vi "echo control.vi"(7 "Read buffer":string="?01E70581\r", 8 "error in":errorcluster) -> (0 "error out":errorcluster, 1 "Сообщение об ошибке":bool, 4 "read buffer wo echo":string, 5 "Ошибка пакета?":bool)   [LabVIEW 2017, in "LV_Unicorn.lvlib"]
uses:
  LV_Unicorn.lvlib
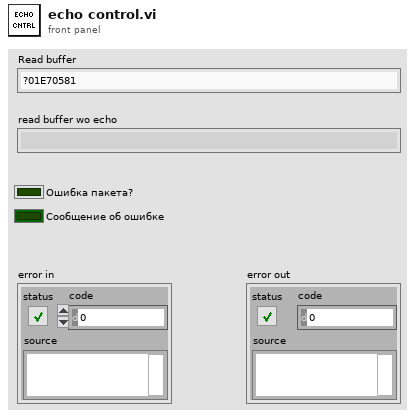
[diagram p1: front panel]
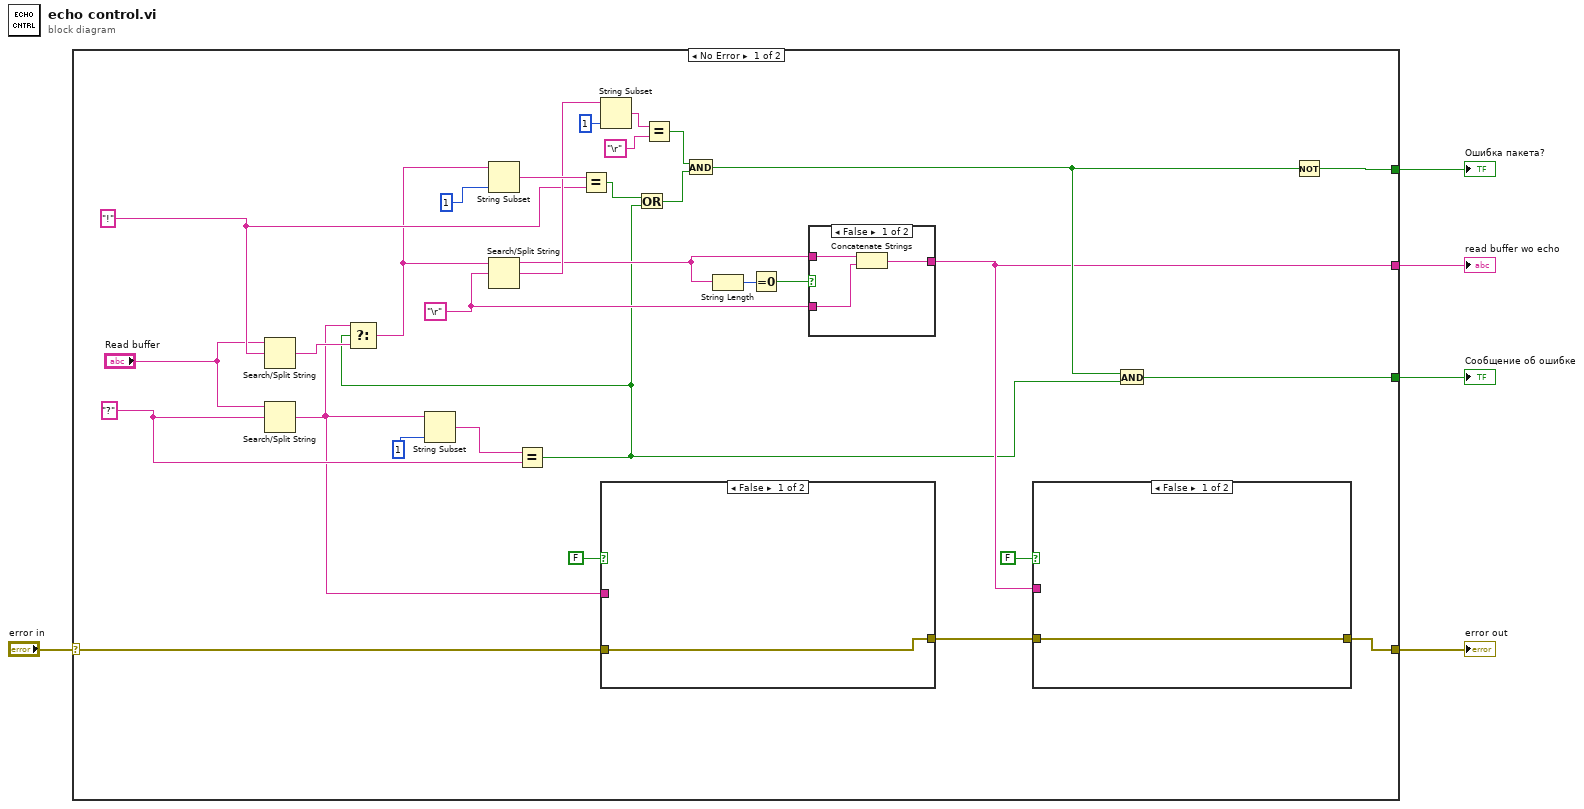
[diagram p0: block diagram]
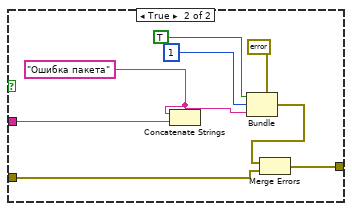
[diagram p2: hidden frame]
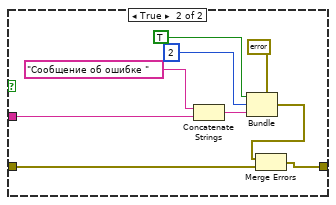
[diagram p3: hidden frame]
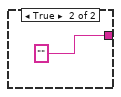
[diagram p4: hidden frame]
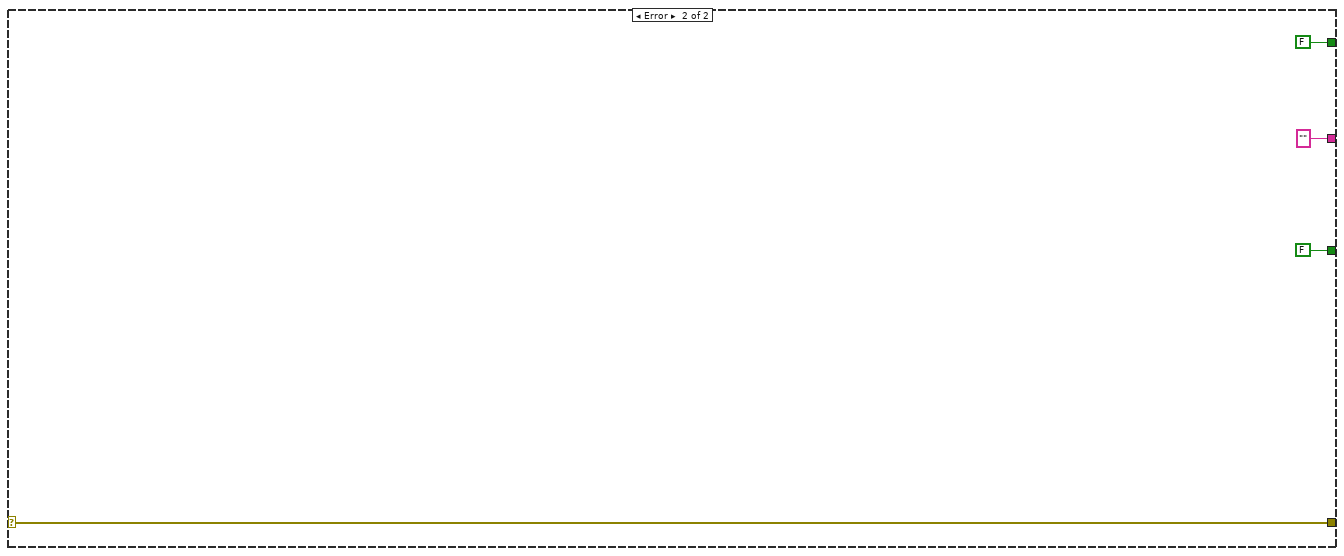
[diagram p5: hidden frame]
diagram:
  n1 = case shown="No Error" "error in" {
    selector: "error in" -> [w7 w63]
    tunnel: [w15 FALSE] -> w5
    tunnel: [w14 w63] -> w4
    tunnel: [w13 ""] -> w3
    tunnel: [w12 FALSE] -> w2
    frame No Error {
      w23 = "?" ("search string/char (-)")
      w21 = "\r" ("search string/char (-)")
      w26 = "!" ("search string/char (-)")
      n2 = Search/Split String(string="Read buffer", search string/char (-)=w26) -> (match + rest of string=w20:string)  [unwired: 1 in, 2 out]
      n3 = Search/Split String(string="Read buffer", search string/char (-)=w23) -> (match + rest of string=w10:string)  [unwired: 1 in, 2 out]
      n4 = String Subset(string=w10, length (rest)=1 ("length (rest)")) -> (substring=w24:string)  [unwired: 1 in]
      n5 = Equal?(x=w24, y=w23) -> (x = y?=w9:bool)
      n6 = Select(t=w10, s=w9, f=w20) -> (s? t:f=w19:string)
      n7 = String Subset(string=w19, length (rest)=1 ("length (rest)")) -> (substring=w34:string)  [unwired: 1 in]
      n8 = Search/Split String(string=w19, search string/char (-)=w21) -> (substring before match=w29:string, match + rest of string=w30:string)  [unwired: 1 in, 1 out]
      n9 = Equal?(x=w34, y=w26) -> (x = y?=w18:bool)
      n10 = String Subset(string=w30, length (rest)=1 ("length (rest)")) -> (substring=w33:string)  [unwired: 1 in]
      n11 = case shown="False" FALSE {
        tunnel: [w37 w42] -> w11
        tunnel: w7 -> [w37 w40]
        tunnel: w10 -> [_ w38]
        frame False {
        }
        frame True {
          w39 = "Ошибка пакета" ("Source")
          n12 = Concatenate Strings(w39, w38) -> ()  [unwired: 1 out]
          n13 = Bundle(cluster=errorcluster {"status"=FALSE, "code"=0, "source"=""} ("error out"), "status"=TRUE, "code"=1 ("Code"), "source"=w39) -> (w41:errorcluster)
          n14 = Merge Errors(w41, w40) -> (w42:errorcluster)
        }
      }
      n15 = Or(x=w18, y=w9) -> (x .or. y?=w17:bool)
      n16 = Equal?(x=w33, y="\r") -> (x = y?=w31:bool)
      n17 = And(x=w31, y=w17) -> (x .and. y?=w16:bool)
      n18 = String Length(string=w29) -> (length=w28:i32)
      n19 = Equal To 0?(x=w28) -> (x = 0?=w27:bool)
      n20 = case shown="False" w27 {
        tunnel: w21 -> [w58 _]
        tunnel: w29 -> [w57 _]
        tunnel: [w56 ""] -> w13
        frame False {
          n21 = Concatenate Strings(w57, w58) -> (w56:string)
        }
        frame True {
        }
      }
      n22 = case shown="False" FALSE {
        tunnel: [w46 w50] -> w14
        tunnel: w13 -> [_ w48]
        tunnel: w11 -> [w46 w47]
        frame False {
        }
        frame True {
          n23 = Concatenate Strings("Сообщение об ошибке " ("Source"), w48) -> (w52:string)
          n24 = Bundle(cluster=errorcluster {"status"=FALSE, "code"=0, "source"=""} ("error out"), "status"=TRUE, "code"=2 ("Code"), "source"=w52) -> (w49:errorcluster)
          n25 = Merge Errors(w49, w47) -> (w50:errorcluster)
        }
      }
      n26 = And(x=w16, y=w9) -> (x .and. y?=w15:bool)
      n27 = Not(x=w16) -> (.not. x?=w12:bool)
    }
    frame Error {
    }
  }
  "read buffer wo echo" <- w3
  "Ошибка пакета?" <- w2
  "Сообщение об ошибке" <- w5
  "error out" <- w4
